vi "ESTTL_Pulse_Gen.vi"(0 "Channel Enable 1":bool, 1 "Channel Enable 2":bool, 2 "Channel Enable 3":bool, 3 "Channel Enable 4":bool, 4 "Channel Enable 5":bool, 5 "Channel Enable 6":bool, 6 "Channel Enable 7":bool, 7 "Channel Enable 8":bool, 8 "ESTTL_Config":T3, 10 "FuelSparkSupervisor":T2, 12 "CmdSequenceChannelSelect":u8, 14 "ESTTL Sequence":T1, 16 "key":u16) -> (20 "CmdOut1":bool, 21 "CmdOut2":bool, 22 "CmdOut3":bool, 23 "CmdOut4":bool, 24 "CmdOut5":bool, 25 "CmdOut6":bool, 26 "CmdOut7":bool, 27 "CmdOut8":bool)   [LabVIEW 2015, in "ECS-FPGA.lvlib"]
uses:
  ECS-FPGA.lvlib
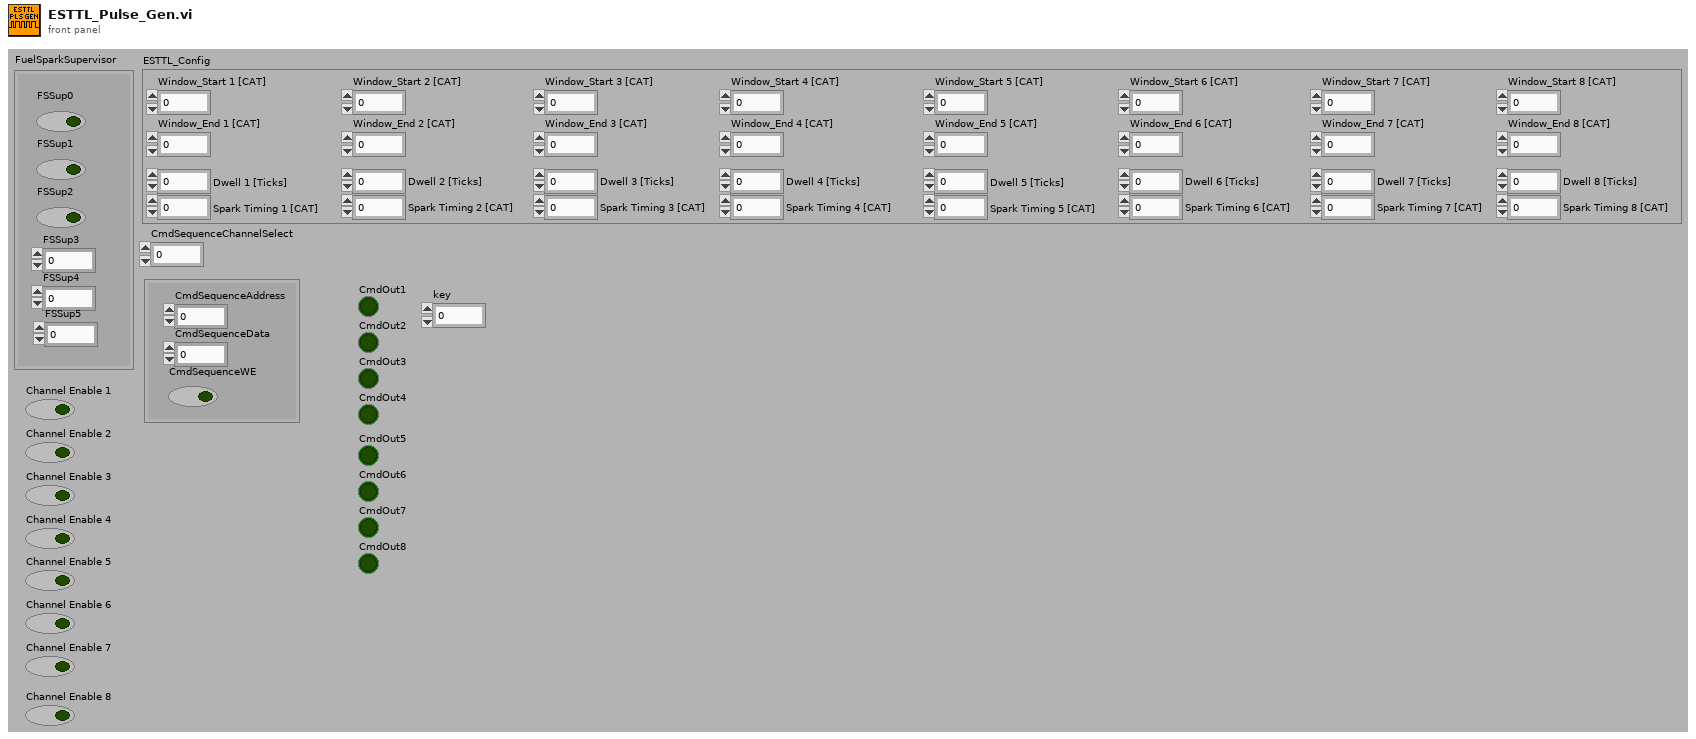
[diagram p1: front panel]
types:
  T1 = cluster{"CmdSequenceAddress":u8, "CmdSequenceData":u32, "CmdSequenceWE":bool}
  T2 = cluster{"FSSup0":bool, "FSSup1":bool, "FSSup2":bool, "FSSup3":u16, "FSSup4":u32, "FSSup5":u16}
  T3 = cluster{"Window_Start 1 [CAT]":u16, "Window_End 1 [CAT]":u16, "Window_Start 2 [CAT]":u16, "Window_End 2 [CAT]":u16, "Window_Start 3 [CAT]":u16, "Window_End 3 [CAT]":u16, "Window_Start 4 [CAT]":u16, "Window_End 4 [CAT]":u16, "Dwell 1 [Ticks]":u32, "Spark Timing 1 [CAT]":u16, "Dwell 2 [Ticks]":u32, "Spark Timing 2 [CAT]":u16, "Dwell 3 [Ticks]":u32, "Spark Timing 3 [CAT]":u16, "Dwell 4 [Ticks]":u32, "Spark Timing 4 [CAT]":u16, "Window_End 5 [CAT]":u16, "Window_Start 5 [CAT]":u16, "Window_End 6 [CAT]":u16, "Window_Start 6 [CAT]":u16, "Window_End 7 [CAT]":u16, "Window_Start 7 [CAT]":u16, "Spark Timing 5 [CAT]":u16, "Dwell 5 [Ticks]":u32, "Spark Timing 6 [CAT]":u16, "Dwell 6 [Ticks]":u32, "Spark Timing 7 [CAT]":u16, "Dwell 7 [Ticks]":u32, "Window_End 8 [CAT]":u16, "Window_Start 8 [CAT]":u16, "Spark Timing 8 [CAT]":u16, "Dwell 8 [Ticks]":u32}
  T4 = cluster{"Enable":bool, "OSAdvance":u32, "OSPosition":u16}
  T5 = cluster{"Enable":bool, "StartPosition":u16, "EndPosition":u16}
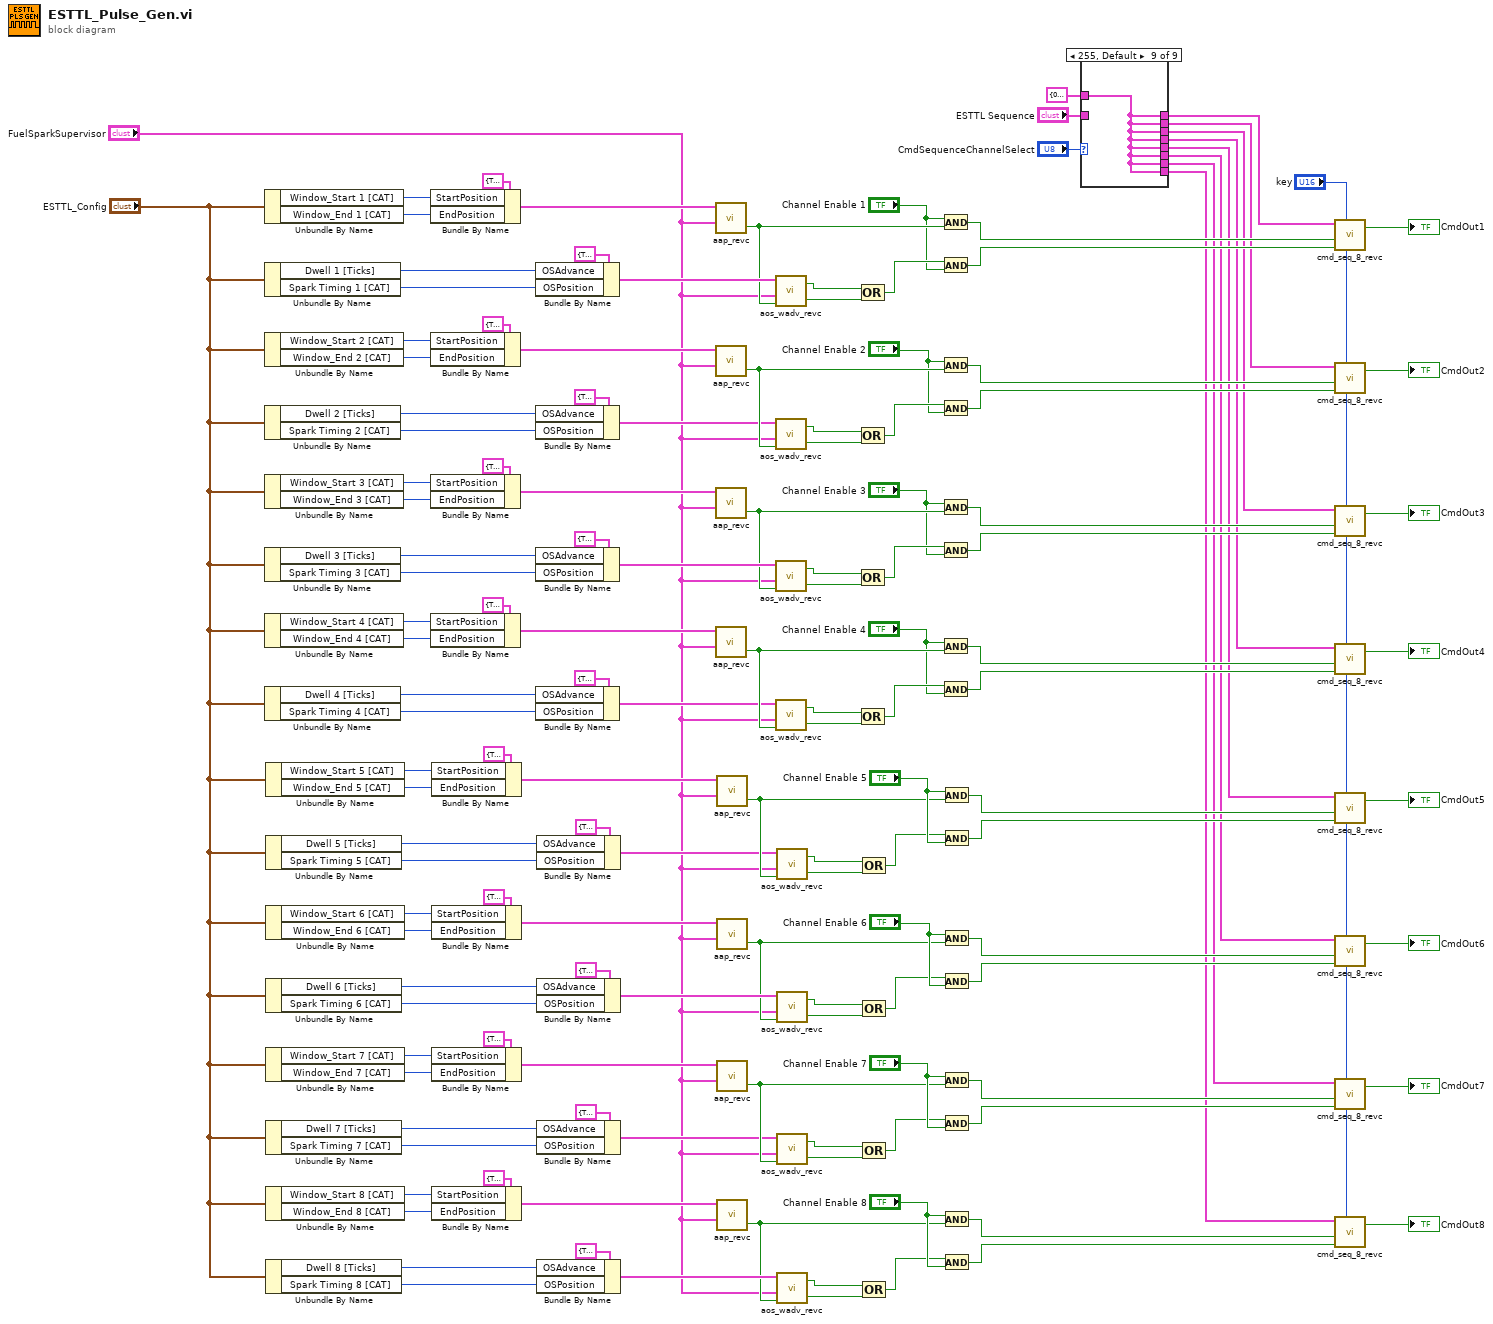
[diagram p0: block diagram]
diagram:
  n1 = Unbundle By Name("ESTTL_Config") -> ("Window_Start 1 [CAT]"=w139:u16, "Window_End 1 [CAT]"=w138:u16)
  n2 = Unbundle By Name("ESTTL_Config") -> ("Dwell 1 [Ticks]"=w136:u32, "Spark Timing 1 [CAT]"=w132:u16)
  n3 = Unbundle By Name("ESTTL_Config") -> ("Window_Start 2 [CAT]"=w125:u16, "Window_End 2 [CAT]"=w126:u16)
  n4 = Unbundle By Name("ESTTL_Config") -> ("Dwell 2 [Ticks]"=w128:u32, "Spark Timing 2 [CAT]"=w131:u16)
  n5 = Unbundle By Name("ESTTL_Config") -> ("Window_Start 3 [CAT]"=w117:u16, "Window_End 3 [CAT]"=w116:u16)
  n6 = Unbundle By Name("ESTTL_Config") -> ("Dwell 3 [Ticks]"=w114:u32, "Spark Timing 3 [CAT]"=w111:u16)
  n7 = Unbundle By Name("ESTTL_Config") -> ("Window_Start 4 [CAT]"=w103:u16, "Window_End 4 [CAT]"=w104:u16)
  n8 = Unbundle By Name("ESTTL_Config") -> ("Dwell 4 [Ticks]"=w106:u32, "Spark Timing 4 [CAT]"=w109:u16)
  n9 = Unbundle By Name("ESTTL_Config") -> ("Window_Start 5 [CAT]"=w18:u16, "Window_End 5 [CAT]"=w19:u16)
  n10 = Unbundle By Name("ESTTL_Config") -> ("Dwell 5 [Ticks]"=w21:u32, "Spark Timing 5 [CAT]"=w25:u16)
  n11 = Unbundle By Name("ESTTL_Config") -> ("Window_Start 6 [CAT]"=w32:u16, "Window_End 6 [CAT]"=w31:u16)
  n12 = Unbundle By Name("ESTTL_Config") -> ("Dwell 6 [Ticks]"=w29:u32, "Spark Timing 6 [CAT]"=w26:u16)
  n13 = Unbundle By Name("ESTTL_Config") -> ("Window_Start 7 [CAT]"=w40:u16, "Window_End 7 [CAT]"=w41:u16)
  n14 = Unbundle By Name("ESTTL_Config") -> ("Dwell 7 [Ticks]"=w43:u32, "Spark Timing 7 [CAT]"=w46:u16)
  n15 = Unbundle By Name("ESTTL_Config") -> ("Window_Start 8 [CAT]"=w54:u16, "Window_End 8 [CAT]"=w53:u16)
  n16 = Unbundle By Name("ESTTL_Config") -> ("Dwell 8 [Ticks]"=w51:u32, "Spark Timing 8 [CAT]"=w48:u16)
  n17 = Bundle By Name(cluster=T5 {"Enable"=TRUE, "StartPosition"=0, "EndPosition"=0} ("OP Windiw Definition"), "StartPosition"=w139, "EndPosition"=w138) -> (w141:T5)
  n18 = Bundle By Name(cluster=T5 {"Enable"=TRUE, "StartPosition"=0, "EndPosition"=0} ("OP Windiw Definition"), "StartPosition"=w125, "EndPosition"=w126) -> (w123:T5)
  n19 = Bundle By Name(cluster=T5 {"Enable"=TRUE, "StartPosition"=0, "EndPosition"=0} ("OP Windiw Definition"), "StartPosition"=w117, "EndPosition"=w116) -> (w119:T5)
  n20 = Bundle By Name(cluster=T5 {"Enable"=TRUE, "StartPosition"=0, "EndPosition"=0} ("OP Windiw Definition"), "StartPosition"=w103, "EndPosition"=w104) -> (w101:T5)
  n21 = Bundle By Name(cluster=T5 {"Enable"=TRUE, "StartPosition"=0, "EndPosition"=0} ("OP Windiw Definition"), "StartPosition"=w18, "EndPosition"=w19) -> (w16:T5)
  n22 = Bundle By Name(cluster=T5 {"Enable"=TRUE, "StartPosition"=0, "EndPosition"=0} ("OP Windiw Definition"), "StartPosition"=w32, "EndPosition"=w31) -> (w34:T5)
  n23 = Bundle By Name(cluster=T5 {"Enable"=TRUE, "StartPosition"=0, "EndPosition"=0} ("OP Windiw Definition"), "StartPosition"=w40, "EndPosition"=w41) -> (w38:T5)
  n24 = Bundle By Name(cluster=T5 {"Enable"=TRUE, "StartPosition"=0, "EndPosition"=0} ("OP Windiw Definition"), "StartPosition"=w54, "EndPosition"=w53) -> (w56:T5)
  n25 = Bundle By Name(cluster=T4 {"Enable"=TRUE, "OSAdvance"=0, "OSPosition"=0} ("AOSControl"), "OSAdvance"=w136, "OSPosition"=w132) -> (w142:T4)
  n26 = Bundle By Name(cluster=T4 {"Enable"=TRUE, "OSAdvance"=0, "OSPosition"=0} ("AOSControl"), "OSAdvance"=w128, "OSPosition"=w131) -> (w122:T4)
  n27 = Bundle By Name(cluster=T4 {"Enable"=TRUE, "OSAdvance"=0, "OSPosition"=0} ("AOSControl"), "OSAdvance"=w114, "OSPosition"=w111) -> (w120:T4)
  n28 = Bundle By Name(cluster=T4 {"Enable"=TRUE, "OSAdvance"=0, "OSPosition"=0} ("AOSControl"), "OSAdvance"=w106, "OSPosition"=w109) -> (w100:T4)
  n29 = Bundle By Name(cluster=T4 {"Enable"=TRUE, "OSAdvance"=0, "OSPosition"=0} ("AOSControl"), "OSAdvance"=w21, "OSPosition"=w25) -> (w15:T4)
  n30 = Bundle By Name(cluster=T4 {"Enable"=TRUE, "OSAdvance"=0, "OSPosition"=0} ("AOSControl"), "OSAdvance"=w29, "OSPosition"=w26) -> (w35:T4)
  n31 = Bundle By Name(cluster=T4 {"Enable"=TRUE, "OSAdvance"=0, "OSPosition"=0} ("AOSControl"), "OSAdvance"=w43, "OSPosition"=w46) -> (w37:T4)
  n32 = Bundle By Name(cluster=T4 {"Enable"=TRUE, "OSAdvance"=0, "OSPosition"=0} ("AOSControl"), "OSAdvance"=w51, "OSPosition"=w48) -> (w57:T4)
  n33 = call <vilib>:"aap_revc.vi"("FuelSparkSupervisor"="FuelSparkSupervisor", "AAPControl"=w141) -> ("AAP"=w135:bool)  [unwired: 3 in]
  n34 = call <vilib>:"aap_revc.vi"("FuelSparkSupervisor"="FuelSparkSupervisor", "AAPControl"=w123) -> ("AAP"=w129:bool)  [unwired: 3 in]
  n35 = call <vilib>:"aap_revc.vi"("FuelSparkSupervisor"="FuelSparkSupervisor", "AAPControl"=w119) -> ("AAP"=w113:bool)  [unwired: 3 in]
  n36 = call <vilib>:"aap_revc.vi"("FuelSparkSupervisor"="FuelSparkSupervisor", "AAPControl"=w101) -> ("AAP"=w107:bool)  [unwired: 3 in]
  n37 = call <vilib>:"aap_revc.vi"("FuelSparkSupervisor"="FuelSparkSupervisor", "AAPControl"=w16) -> ("AAP"=w22:bool)  [unwired: 3 in]
  n38 = call <vilib>:"aap_revc.vi"("FuelSparkSupervisor"="FuelSparkSupervisor", "AAPControl"=w34) -> ("AAP"=w28:bool)  [unwired: 3 in]
  n39 = call <vilib>:"aap_revc.vi"("FuelSparkSupervisor"="FuelSparkSupervisor", "AAPControl"=w38) -> ("AAP"=w44:bool)  [unwired: 3 in]
  n40 = call <vilib>:"aap_revc.vi"("FuelSparkSupervisor"="FuelSparkSupervisor", "AAPControl"=w56) -> ("AAP"=w50:bool)  [unwired: 3 in]
  n41 = call <vilib>:"aos_wadv_revc.vi"("OpWindow"=w135, "FuelSparkSupervisor"="FuelSparkSupervisor", "AOSControl"=w142) -> ("AOS"=w82:bool, "AOSAdv"=w86:bool)  [unwired: 1 in]
  n42 = call <vilib>:"aos_wadv_revc.vi"("OpWindow"=w129, "FuelSparkSupervisor"="FuelSparkSupervisor", "AOSControl"=w122) -> ("AOS"=w81:bool, "AOSAdv"=w85:bool)  [unwired: 1 in]
  n43 = call <vilib>:"aos_wadv_revc.vi"("OpWindow"=w113, "FuelSparkSupervisor"="FuelSparkSupervisor", "AOSControl"=w120) -> ("AOS"=w80:bool, "AOSAdv"=w84:bool)  [unwired: 1 in]
  n44 = call <vilib>:"aos_wadv_revc.vi"("OpWindow"=w107, "FuelSparkSupervisor"="FuelSparkSupervisor", "AOSControl"=w100) -> ("AOS"=w79:bool, "AOSAdv"=w83:bool)  [unwired: 1 in]
  n45 = call <vilib>:"aos_wadv_revc.vi"("OpWindow"=w22, "FuelSparkSupervisor"="FuelSparkSupervisor", "AOSControl"=w15) -> ("AOS"=w75:bool, "AOSAdv"=w71:bool)  [unwired: 1 in]
  n46 = call <vilib>:"aos_wadv_revc.vi"("OpWindow"=w28, "FuelSparkSupervisor"="FuelSparkSupervisor", "AOSControl"=w35) -> ("AOS"=w76:bool, "AOSAdv"=w72:bool)  [unwired: 1 in]
  n47 = call <vilib>:"aos_wadv_revc.vi"("OpWindow"=w44, "FuelSparkSupervisor"="FuelSparkSupervisor", "AOSControl"=w37) -> ("AOS"=w77:bool, "AOSAdv"=w73:bool)  [unwired: 1 in]
  n48 = call <vilib>:"aos_wadv_revc.vi"("OpWindow"=w50, "FuelSparkSupervisor"="FuelSparkSupervisor", "AOSControl"=w57) -> ("AOS"=w78:bool, "AOSAdv"=w74:bool)  [unwired: 1 in]
  n49 = Compound Arithmetic op=OR(w86, w82) -> (w137:bool)
  n50 = Compound Arithmetic op=OR(w85, w81) -> (w127:bool)
  n51 = Compound Arithmetic op=OR(w84, w80) -> (w115:bool)
  n52 = Compound Arithmetic op=OR(w83, w79) -> (w105:bool)
  n53 = Compound Arithmetic op=OR(w71, w75) -> (w20:bool)
  n54 = Compound Arithmetic op=OR(w72, w76) -> (w30:bool)
  n55 = Compound Arithmetic op=OR(w73, w77) -> (w42:bool)
  n56 = Compound Arithmetic op=OR(w74, w78) -> (w52:bool)
  n57 = And(x="Channel Enable 1", y=w135) -> (x .and. y?=w97:bool)
  n58 = And(x=w137, y="Channel Enable 1") -> (x .and. y?=w98:bool)
  n59 = And(x="Channel Enable 2", y=w129) -> (x .and. y?=w95:bool)
  n60 = And(x=w127, y="Channel Enable 2") -> (x .and. y?=w94:bool)
  n61 = And(x="Channel Enable 3", y=w113) -> (x .and. y?=w92:bool)
  n62 = And(x=w115, y="Channel Enable 3") -> (x .and. y?=w91:bool)
  n63 = And(x="Channel Enable 4", y=w107) -> (x .and. y?=w89:bool)
  n64 = And(x=w105, y="Channel Enable 4") -> (x .and. y?=w88:bool)
  n65 = And(x="Channel Enable 5", y=w22) -> (x .and. y?=w60:bool)
  n66 = And(x=w20, y="Channel Enable 5") -> (x .and. y?=w59:bool)
  n67 = And(x="Channel Enable 6", y=w28) -> (x .and. y?=w62:bool)
  n68 = And(x=w30, y="Channel Enable 6") -> (x .and. y?=w63:bool)
  n69 = And(x="Channel Enable 7", y=w44) -> (x .and. y?=w65:bool)
  n70 = And(x=w42, y="Channel Enable 7") -> (x .and. y?=w66:bool)
  n71 = And(x="Channel Enable 8", y=w50) -> (x .and. y?=w68:bool)
  n72 = And(x=w52, y="Channel Enable 8") -> (x .and. y?=w69:bool)
  n73 = case shown="255, Default" "CmdSequenceChannelSelect" {
    tunnel: "ESTTL Sequence" -> [w143 w145 w148 w150 w152 w154 w156 w158 _]
    tunnel: [w143 w146 w147 w149 w151 w153 w155 w157 w159] -> w9
    tunnel: [w144 w145 w147 w149 w151 w153 w155 w157 w159] -> w8
    tunnel: [w144 w146 w148 w149 w151 w153 w155 w157 w159] -> w7
    tunnel: [w144 w146 w147 w150 w151 w153 w155 w157 w159] -> w6
    tunnel: [w144 w146 w147 w149 w152 w153 w155 w157 w159] -> w5
    tunnel: [w144 w146 w147 w149 w151 w154 w155 w157 w159] -> w4
    tunnel: [w144 w146 w147 w149 w151 w153 w156 w157 w159] -> w3
    tunnel: [w144 w146 w147 w149 w151 w153 w155 w158 w159] -> w2
    tunnel: T1 {"CmdSequenceAddress"=0, "CmdSequenceData"=0, "CmdSequenceWE"=FALSE} ("ESTTL Sequence") -> [w144 w146 w147 w149 w151 w153 w155 w157 w159]
    frame 0 {
    }
    frame 1 {
    }
    frame 2 {
    }
    frame 3 {
    }
    frame 4 {
    }
    frame 5 {
    }
    frame 6 {
    }
    frame 7 {
    }
    frame 255, Default {
    }
  }
  n74 = call <vilib>:"cmd_seq_8_revc.vi"("CmdSequencePort"=w9, "SequenceReset"=w97, "Trigger"=w98, "key"="key") -> ("Command"=→"CmdOut1":bool)  [unwired: 1 in, 1 out]
  n75 = call <vilib>:"cmd_seq_8_revc.vi"("CmdSequencePort"=w8, "SequenceReset"=w95, "Trigger"=w94, "key"="key") -> ("Command"=→"CmdOut2":bool)  [unwired: 1 in, 1 out]
  n76 = call <vilib>:"cmd_seq_8_revc.vi"("CmdSequencePort"=w7, "SequenceReset"=w92, "Trigger"=w91, "key"="key") -> ("Command"=→"CmdOut3":bool)  [unwired: 1 in, 1 out]
  n77 = call <vilib>:"cmd_seq_8_revc.vi"("CmdSequencePort"=w6, "SequenceReset"=w89, "Trigger"=w88, "key"="key") -> ("Command"=→"CmdOut4":bool)  [unwired: 1 in, 1 out]
  n78 = call <vilib>:"cmd_seq_8_revc.vi"("CmdSequencePort"=w5, "SequenceReset"=w60, "Trigger"=w59, "key"="key") -> ("Command"=→"CmdOut5":bool)  [unwired: 1 in, 1 out]
  n79 = call <vilib>:"cmd_seq_8_revc.vi"("CmdSequencePort"=w4, "SequenceReset"=w62, "Trigger"=w63, "key"="key") -> ("Command"=→"CmdOut6":bool)  [unwired: 1 in, 1 out]
  n80 = call <vilib>:"cmd_seq_8_revc.vi"("CmdSequencePort"=w3, "SequenceReset"=w65, "Trigger"=w66, "key"="key") -> ("Command"=→"CmdOut7":bool)  [unwired: 1 in, 1 out]
  n81 = call <vilib>:"cmd_seq_8_revc.vi"("CmdSequencePort"=w2, "SequenceReset"=w68, "Trigger"=w69, "key"="key") -> ("Command"=→"CmdOut8":bool)  [unwired: 1 in, 1 out]
